vi "save_sweep.vi"(7 "sweep index":i32, 8 "error in (no error)":errorcluster, 9 "base name":string, 10 "folder path":path, 11 "DataCollectionMG091001IntrinsicImaging in":refnum<class "DataCollectionMG091001IntrinsicImaging.lvclass">) -> (0 "error out":errorcluster, 3 "DataCollectionMG091001IntrinsicImaging out":refnum<class "DataCollectionMG091001IntrinsicImaging.lvclass">)   [LabVIEW 2010, in "DataCollectionMG091001IntrinsicImaging.lvclass"]
uses:
  DataCollectionMG091001IntrinsicImaging.lvclass
  sweep_part_enum.ctl
  DataCollectionMG091001IntrinsicImaging.lvclass/DataCollectionMG091001IntrinsicImaging.ctl
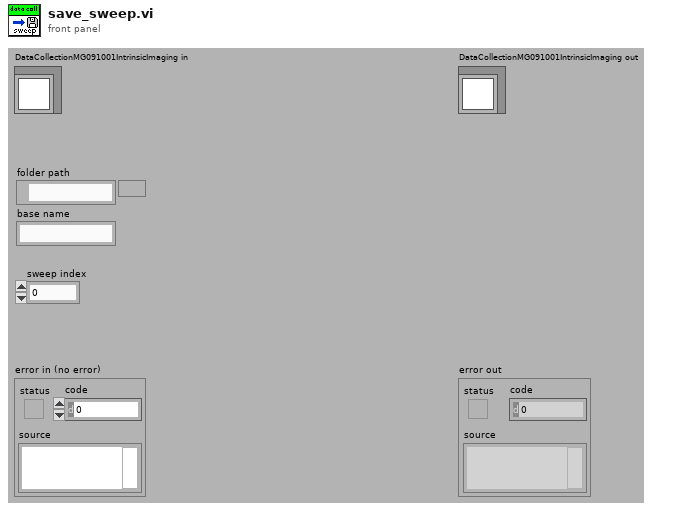
[diagram p1: front panel]
types:
  T1 = typedef "DataCollectionMG091001IntrinsicImaging.lvclass/sweep_part_enum.ctl" = enum16{"actual measurement", "control"}
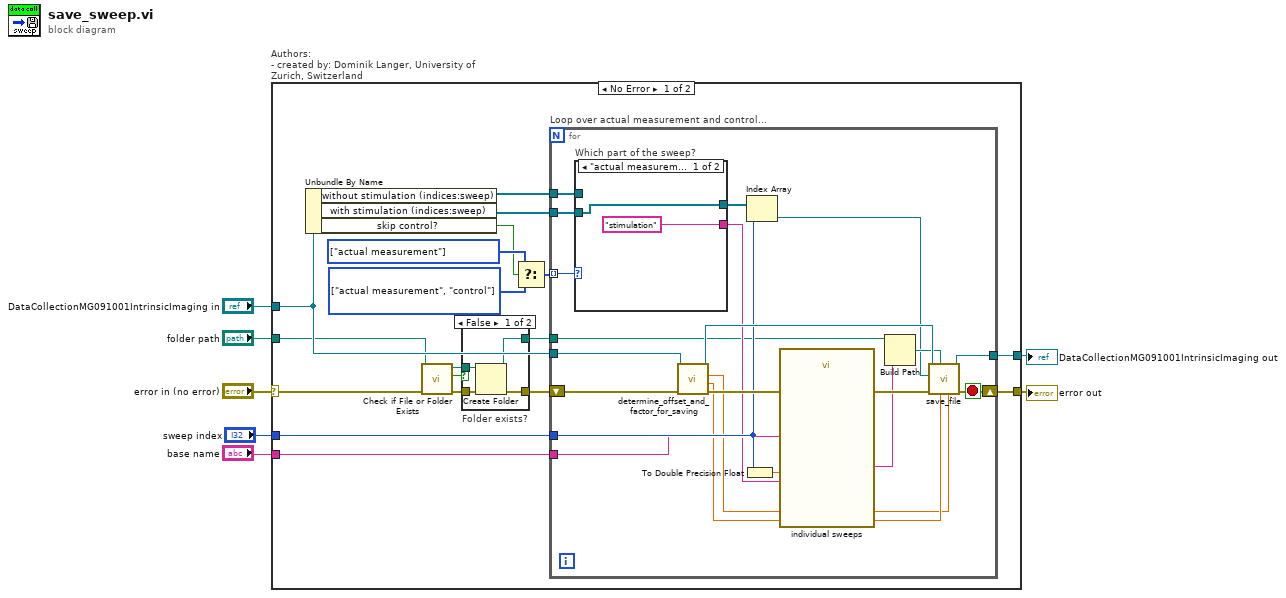
[diagram p0: block diagram]
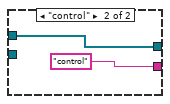
[diagram p3: hidden frame]
diagram:
  n1 = case "Authors: \n- created by: Dominik Langer, University of Zurich, Switzerland" shown="No Error" "error in (no error)" {
    selector: "error in (no error)" -> [w8 w58]
    tunnel: [w9 w58] -> w6
    tunnel: [w23 w57] -> w4
    tunnel: "DataCollectionMG091001IntrinsicImaging in" -> [w14 w57]
    tunnel: "folder path" -> [w12 _]
    tunnel: "base name" -> [w15 _]
    tunnel: "sweep index" -> [w22 _]
    frame No Error {
      w20 = T1[] [enum."actual measurement", enum."control"] items=["actual measurement", "control"]
      w21 = T1[] [enum."actual measurement"] items=["actual measurement", "control"]
      n2 = Unbundle By Name(w14) -> ("without stimulation (indices:sweep)"=w25:refnum<class "ImageCollection.lvclass">[], "with stimulation (indices:sweep)"=w24:refnum<class "ImageCollection.lvclass">[], "skip control?"=w19:bool)
      n3 = call <vilib>:"Check if File or Folder Exists.vi"("error in (no error)"=w8, "path"=w12) -> ("error out"=w13:errorcluster, "file or folder exists?"=w10:bool, "dup path"=w11:path)  [unwired: 7 in]
      n4 = case "Folder exists?" shown="False" w10 {
        tunnel: [w29 w31] -> w17
        tunnel: [w28 w30] -> w16
        tunnel: w13 -> [w27 w31]
        tunnel: w11 -> [w26 w30]
        frame False {
          n5 = Create Folder(path (use dialog)=w26, error in=w27) -> (created path=w28:path, error out=w29:errorcluster)  [unwired: 1 in, 1 out]
        }
        frame True {
        }
      }
      n6 = Select(t=w21, s=w19, f=w20) -> (s? t:f=w18:T1[])
      n7 = for "Loop over actual measurement and control..." {
        tunnel: w25 -> [w52]
        tunnel: w24 -> [w51]
        tunnel: w16 -> [w37]
        tunnel: w15 -> [w40]
        tunnel: w14 -> [w47]
        tunnel: [w32] -> w23
        tunnel: w22 -> [w42]
        tunnel: w18 -> [w41] mode=indexing
        shift-right: [w33] -> w9
        shift-left: w17 -> [w48]
        stop <- w33 stop-if-true
        n8 = case "Which part of the sweep?" shown="\"actual measurement\", Default" w41 {
          tunnel: w52 -> [_ w56]
          tunnel: w51 -> [w54 _]
          tunnel: [w54 w56] -> w43
          tunnel: ["stimulation" "control"] -> w38
          frame "actual measurement", Default {
          }
          frame "control" {
          }
        }
        n9 = call-dynamic "determine_offset_and_factor_for_saving.vi"("error in (no error)"=w48, "DataCollectionMG091001IntrinsicImaging in"=w47) -> ("error out"=w49:errorcluster, "factor"=w36:dbl, "offset"=w35:dbl, "DataCollectionMG091001IntrinsicImaging out"=w50:refnum<class "DataCollectionMG091001IntrinsicImaging.lvclass">)  [unwired: 6 in]
        n10 = To Double Precision Float(number=w42) -> (double precision float=w39:dbl)
        n11 = Index Array(array=w43, index=w42) -> (element=w34:refnum<class "ImageCollection.lvclass">)
        n12 = call "individual sweeps"("factor"=w36, "base"=w40, "sweep"=w39, "type"=w38, "error in (no error)"=w49, "offset"=w35) -> ("Result"=w44:string, "error out"=w46:errorcluster)  [unwired: 8 in]
        n13 = Build Path(base path=w37, name or relative path=w44) -> (appended path=w45:path)
        n14 = call-dynamic "save_file.vi"("offset"=w35, "multiplication factor"=w36, "path"=w45, "error in (no error)"=w46, "ImageCollection in"=w34, "DataCollectionDL090215 in"=w50) -> ("error out"=w33:errorcluster, "DataCollectionDL090215 out"=w32:refnum<class "DataCollectionMG091001IntrinsicImaging.lvclass">)  [unwired: 4 in]
      }
    }
    frame Error {
    }
  }
  "error out" <- w6
  "DataCollectionMG091001IntrinsicImaging out" <- w4
